vi "test.vi"() -> ()   [LabVIEW 2019]
panel:
  in  "stop":bool
  in  "x0":dbl(slide) scale=-115.0..115.0
  in  "z0":dbl(slide) scale=-135.0..50.0
  in  "y0":dbl(slide) scale=-115.0..115.0
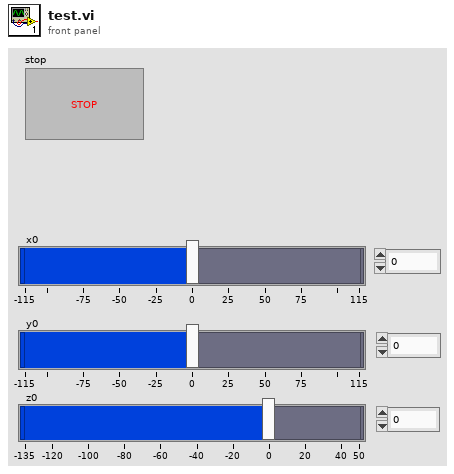
[diagram p1: front panel]
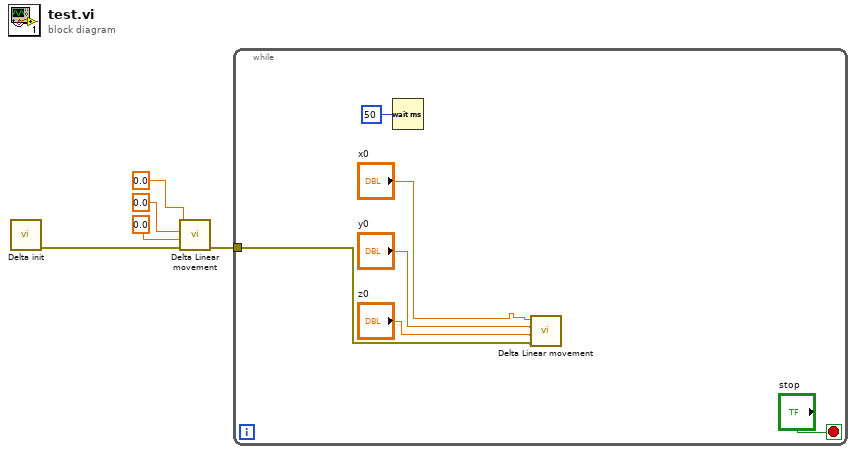
[diagram p0: block diagram]
diagram:
  n1 = call "Delta init.vi"() -> ("error out"=w2:errorcluster)  [unwired: 9 in, 2 out]
  n2 = call "Delta Linear movement.vi"("error in (no error)"=w2, "z0"=0.0, "y0"=0.0, "x0"=0.0) -> ("error out"=w1:errorcluster)  [unwired: 7 in]
  n3 = while {
    tunnel: w1 -> [w10]
    stop <- "stop" stop-if-true
    n4 = Wait (ms)(milliseconds to wait=u32 50) -> ()  [unwired: 1 out]
    n5 = call "Delta Linear movement.vi"("error in (no error)"=w10, "z0"="z0", "y0"="y0", "x0"="x0") -> ()  [unwired: 7 in, 1 out]
  }
